vi "Material-ConfigPage-Initialize.vi"(0 "Configuration Page":refnum<class "Material-ConfigPage.lvclass">, 11 "error in":errorcluster) -> (4 "Configuration Page out":refnum<class "Material-ConfigPage.lvclass">, 15 "error out":errorcluster)   [LabVIEW 2014, in "Material-ConfigPage.lvclass"]
uses:
  Material-ConfigPage.lvclass
  Material-ConfigPage.lvclass/Material-ConfigPage.ctl
  Reuse Library/featherweight/Core/Messaging/Messenger.Actor/FTW-Messenger-Actor.lvclass
  Reuse Library/featherweight/Core/Container/FTW-Container.lvclass
panel:
  # "Inputs"
  # "Outputs"
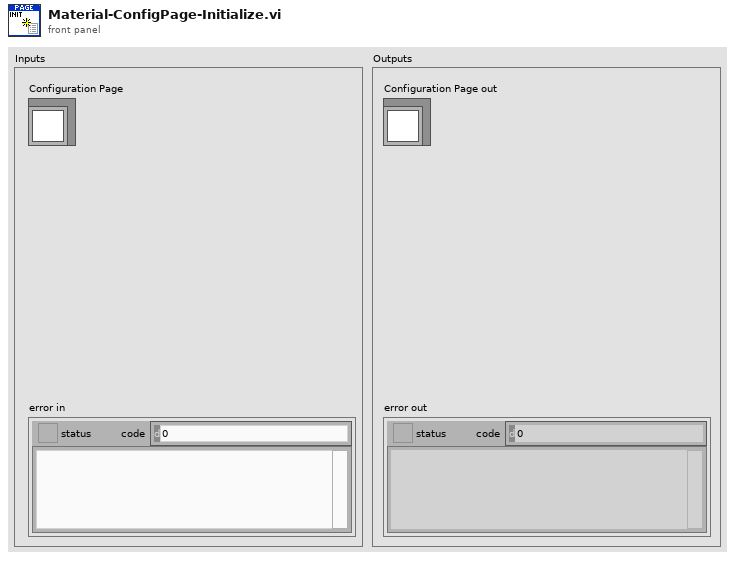
[diagram p1: front panel]
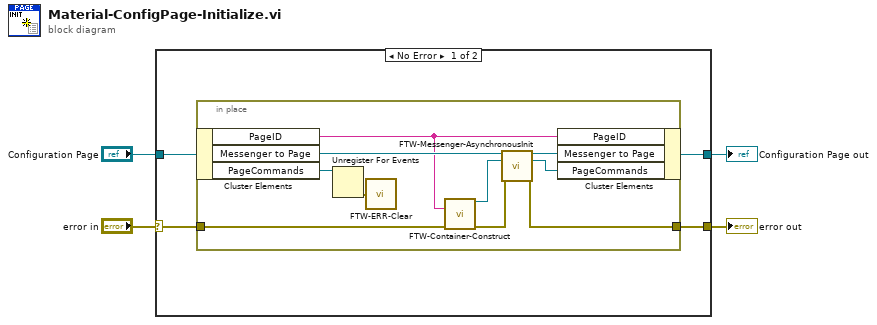
[diagram p0: block diagram]
diagram:
  n1 = case shown="No Error" "error in" {
    selector: "error in" -> [w8 w20]
    tunnel: [w7 w20] -> w4
    tunnel: [w6 w19] -> w2
    tunnel: "Configuration Page" -> [w5 w19]
    frame No Error {
      n2 = in-place {
        in-place-border: w8 -> [w11]
        in-place-border: [w17] -> w7
        n3 = in-place-cluster #1(w5) -> ("PageID"=w9:string, "Messenger to Page"=w18:refnum<class "FTW-Messenger-Actor.lvclass">, "PageCommands"=w15:refnum<event-registration>)
        n4 = Unregister For Events(event registration refnum=w15) -> (error out=w14:errorcluster)  [unwired: 1 in]
        n5 = call "FTW-ERR-Clear.vi"("error to snuff"=w14) -> ()  [unwired: 1 out]
        n6 = call "FTW-Container-Construct.vi"("LabVIEW Data Structure"=w9, "error in"=w11) -> ("Container"=w12:refnum<class "FTW-Container.lvclass">, "error out"=w10:errorcluster)  [unwired: 12 in]
        n7 = call-dynamic "FTW-Messenger-AsynchronousInit.vi"("Messenger"=w18, "Initialized Response"=w12, "error in"=w10) -> ("Initialized Messenger"=w13:refnum<class "FTW-Messenger-Actor.lvclass">, "Observer"=w16:refnum<event-registration>, "error out"=w17:errorcluster)  [unwired: 10 in]
        n8 = in-place-cluster #1("PageID"=w9, "Messenger to Page"=w13, "PageCommands"=w16) -> (w6:refnum<class "Material-ConfigPage.lvclass">)
      }
    }
    frame Error {
    }
  }
  "error out" <- w4
  "Configuration Page out" <- w2
